vi "Actor Core.vi"(8 "error in":errorcluster, 11 "Nested in":refnum<class "SubPanel User Interface.lvclass">) -> (0 "error out":errorcluster, 3 "Actor out":refnum<class "Actor.lvclass">)   [LabVIEW 2015, in "SubPanel User Interface.lvlib" / "SubPanel User Interface.lvclass"]
doc: "(<B>Filename</B>: Actor Framework.lvlib:Actor.lvclass:Actor Core.vi)\n\nReceives messages to the actor, reacts to them, and initiates any error handling that may shut the actor down.\n\nDescendant classes may override this VI to append parallel tasks for the actor to complete while it handles messages. Overrides use the Call Parent Method node."
uses:
  SubPanel User Interface.lvclass
  <vilib>/ActorFramework/Actor/Actor.lvclass
  <vilib>/ActorFramework/Actor/Actor.lvclass/Actor.ctl
  <vilib>/ActorFramework/Message Enqueuer/Message Enqueuer.lvclass/Message Enqueuer.ctl
  SubPanel User Interface.lvclass/SubPanel User Interface.ctl
  SubPanel User Interface Messages/New Panel Selected Msg/New Panel Selected Msg.lvclass/New Panel Selected Msg.ctl
  SubPanel User Interface Messages/Right Click Menu Activated Msg/Right Click Menu Activated Msg.lvclass/Right Click Menu Activated Msg.ctl
  SubPanel User Interface Messages/Right Click Menu Selected Msg/Right Click Menu Selected Msg.lvclass/Right Click Menu Selected Msg.ctl
  <vilib>/ActorFramework/Message Enqueuer/Init from Existing Queue.vi
  <vilib>/ActorFramework/Message Enqueuer/Enqueue.vi
  <vilib>/ActorFramework/Message Priority Queue/Priority Enqueue.vi
  <vilib>/ActorFramework/Message Enqueuer/Message Enqueuer.lvclass
  SubPanel User Interface Messages/New Panel Selected Msg/New Panel Selected Msg.lvclass
  <vilib>/ActorFramework/Stop Msg/Stop Msg.lvclass
  SubPanel User Interface Messages/Right Click Menu Activated Msg/Right Click Menu Activated Msg.lvclass
  SubPanel User Interface Messages/Right Click Menu Selected Msg/Right Click Menu Selected Msg.lvclass
panel:
  in  "Close":bool
  in  "Chat Window":i32(listbox)
  out "Panel":string
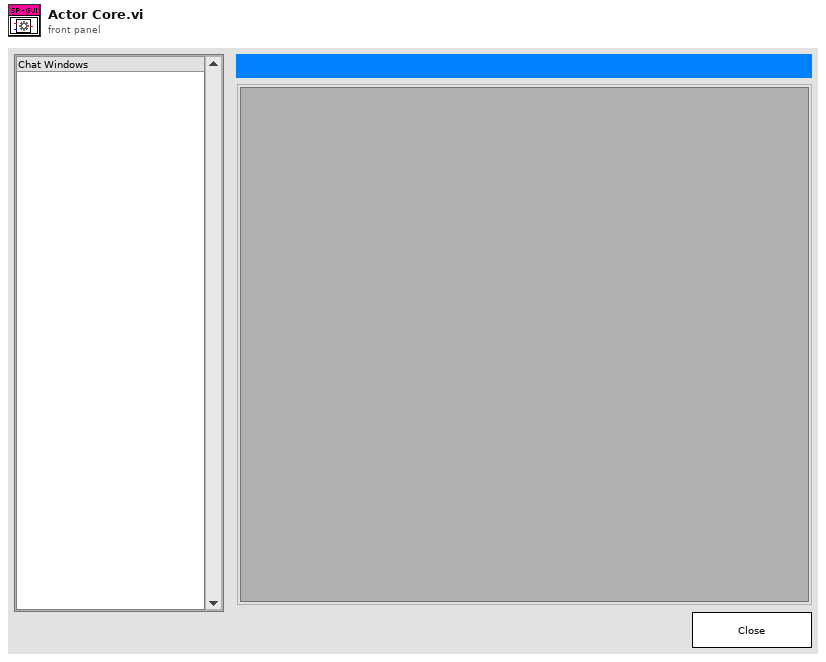
[diagram p1: front panel]
types:
  T1 = cluster{"Stop":refnum<user-event>, "Panel":refnum<user-event>}
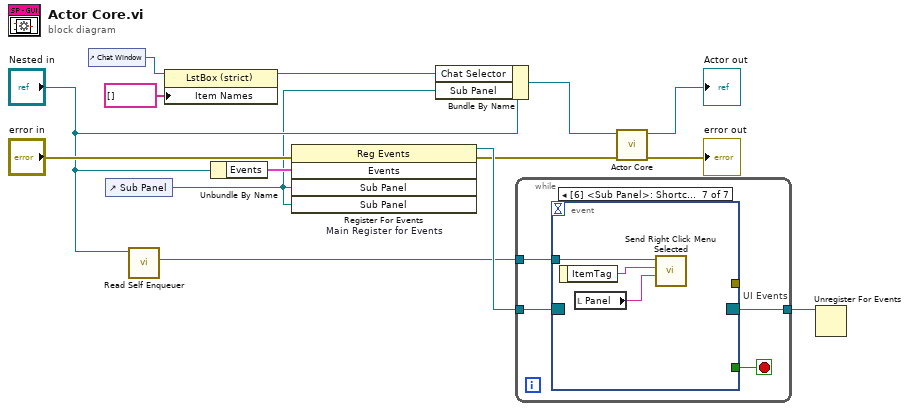
[diagram p0: block diagram]
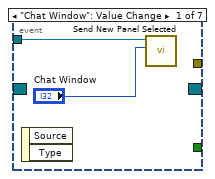
[diagram p2: hidden frame]
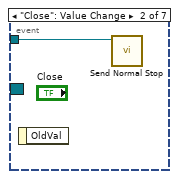
[diagram p3: hidden frame]
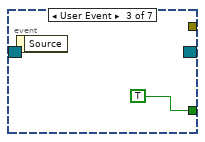
[diagram p4: hidden frame]
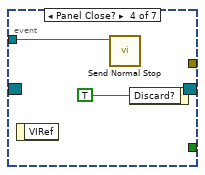
[diagram p5: hidden frame]
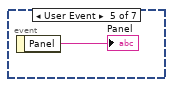
[diagram p6: hidden frame]
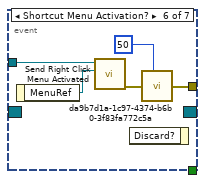
[diagram p7: hidden frame]
diagram:
  n1 = control-ref of="Chat Window"() -> (w3:refnum<vi>)
  n2 = control-ref of="Sub Panel"() -> (w4:refnum<vi>)
  n3 = call <vilib>:"Read Self Enqueuer.vi"("Actor"="Nested in") -> ("Self Enqueuer"=w9:refnum<class "Message Enqueuer.lvclass">)  [unwired: 10 in]
  n4 = property class="LstBox (strict)"(reference=w3, "Item Names"=string[] []) -> (reference out=w2:refnum<vi>)  [unwired: 1 in, 1 out]
  n5 = Unbundle By Name("Nested in") -> ("Events"=w11:T1)
  n6 = register-events "Main Register for Events"(error in="error in", w11, w4, w4) -> (reference out=w12:refnum<event-registration>, error out=w7:errorcluster)  [unwired: 1 in]
  n7 = Bundle By Name(cluster="Nested in", "Chat Selector"=w2, "Sub Panel"=w4) -> (w5:refnum<class "SubPanel User Interface.lvclass">)
  n8 = while {
    tunnel: w12 -> [w18]
    tunnel: [w16] -> w10
    tunnel: w9 -> [w15]
    stop <- w17 stop-if-true
    n9 = event "UI Events" shown="[6] <Sub Panel>: Shortcut Menu Selection (User)" {
      selector: w18 -> [_ _ _ _ _ _ _]
      dyn-events: [_ _ _ _ _ _ _] -> w16
      timeout: _ -> [_ _ _ _ _ _ _]
      tunnel: [_ _ TRUE _ _ _ _] -> w17
      tunnel: w15 -> [w20 w21 _ w23 _ w30 w33]
      tunnel: [_ _ _ _ _ w27 _] -> _
      event "Chat Window": Value Change {
        n10 = event-data() -> ()  [unwired: 1 in, 2 out]
        n11 = call "Send New Panel Selected.vi"("Chat Window"="Chat Window", "Message Enqueuer"=w20) -> ()  [unwired: 8 in, 2 out]
      }
      event "Close": Value Change {
        n12 = event-data() -> ()  [unwired: 1 in, 1 out]
        n13 = call <vilib>:"Send Normal Stop.vi"("Message Enqueuer"=w21) -> ()  [unwired: 10 in, 1 out]
      }
      event User Event {
        n14 = event-data() -> ()  [unwired: 1 in, 1 out]
      }
      event Panel Close? {
        n15 = event-data() -> ()  [unwired: 1 in, 1 out]
        n16 = call <vilib>:"Send Normal Stop.vi"("Message Enqueuer"=w23) -> ()  [unwired: 10 in, 1 out]
        n17 = event-data("Discard?"=TRUE) -> ()  [unwired: 1 in, 1 out]
      }
      event User Event {
        n18 = event-data() -> ("Panel"=→"Panel":string)  [unwired: 1 in]
      }
      event Shortcut Menu Activation? {
        n19 = event-data() -> ("MenuRef"=w29:refnum<k9>)  [unwired: 1 in]
        n20 = call "Send Right Click Menu Activated.vi"("MenuRef"=w29, "Message Enqueuer"=w30) -> ("error out"=w28:errorcluster)  [unwired: 8 in, 1 out]
        n21 = event-data() -> ()  [unwired: 2 in, 1 out]
        n22 = call "da9b7d1a-1c97-4374-b6b0-3f83fa772c5a.vi"("value in"=w28, "milliseconds to wait"=u32 50) -> ("value out"=w27:errorcluster)  [unwired: 1 out]
      }
      event Shortcut Menu Selection (User) {
        n23 = event-data() -> ("ItemTag"=w32:string)  [unwired: 1 in]
        n24 = local read "Panel"() -> (w31:string)
        n25 = call "Send Right Click Menu Selected.vi"("Panel"=w31, "Tag"=w32, "Message Enqueuer"=w33) -> ()  [unwired: 7 in, 2 out]
      }
    }
  }
  n26 = call-parent "Actor Core.vi"("error in"=w7, "Actor in"=w5) -> ("error out"=→"error out":errorcluster, "Actor out"=→"Actor out":refnum<class "Actor.lvclass">)  [unwired: 8 in]
  n27 = Unregister For Events(event registration refnum=w10) -> ()  [unwired: 1 in, 1 out]
